vi "LaserCal-Initialize (Dynamic).vi"(0 "Dynamic I-O Params":T1={"Vcommand"="1:0.5:3", "Repeats"=0, "Scramble"=FALSE}, 5 "Taverage (ms)":dbl, 11 "error in (no error)":errorcluster) -> (2 "Stimulus":T4, 4 "Runtime State":T3={"AO Channels"=[], "Fs (Hz)"=100000.0, "Npts"=1}, 8 "SeqVars":dbl[](array[numeric]), 14 "I-O Data":T2, 15 "error out":errorcluster)   [LabVIEW 2015]
uses:
  Typedefs/LaserCal-Stimulus Params.ctl
  Typedefs/LaserCal-Meter Runtime State.ctl
  Typedefs/LaserCal-Data (Dynamic).ctl
  Typedefs/LaserCal-Dynamic I-O Params.ctl
  <vilib>/Analysis/1siggen.llb/Riffle Array (DBL).vi
  <vilib>/Analysis/NI_AALBase.lvlib
panel:
  in  "Fs (Hz)":dbl=100000.0
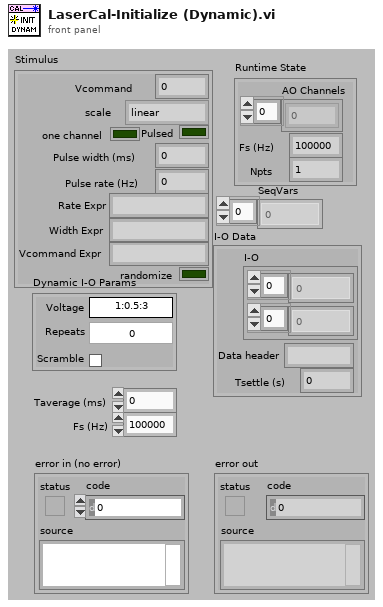
[diagram p1: front panel]
types:
  T1 = typedef "LaserCal-Dynamic I-O Params.ctl" = cluster{"Vcommand":string, "Repeats":i32, "Scramble":bool}
  T2 = typedef "LaserCal-Data (Dynamic).ctl" = cluster{"I-O":cluster{dbl[], dbl[]}, "Data header":string, "Tsettle (s)":dbl}
  T3 = typedef "LaserCal-Meter Runtime State.ctl" = cluster{"AO Channels":i32[], "Fs (Hz)":dbl, "Npts":i32}
  T4 = typedef "LaserCal-Stimulus Params.ctl" = cluster{"Vcommand":dbl, "scale":enum16{"linear", "dB"}, "Pulsed":bool, "Pulse width (ms)":dbl, "Pulse rate (Hz)":dbl, "Vcommand Expr":string, "Width Expr":string, "one channel":bool, "Rate Expr":string, "randomize":bool}
  T5 = cluster{cluster{"Riffled {X}":dbl[], dbl[]}, "Header out":string, "Taverage (ms)":dbl}
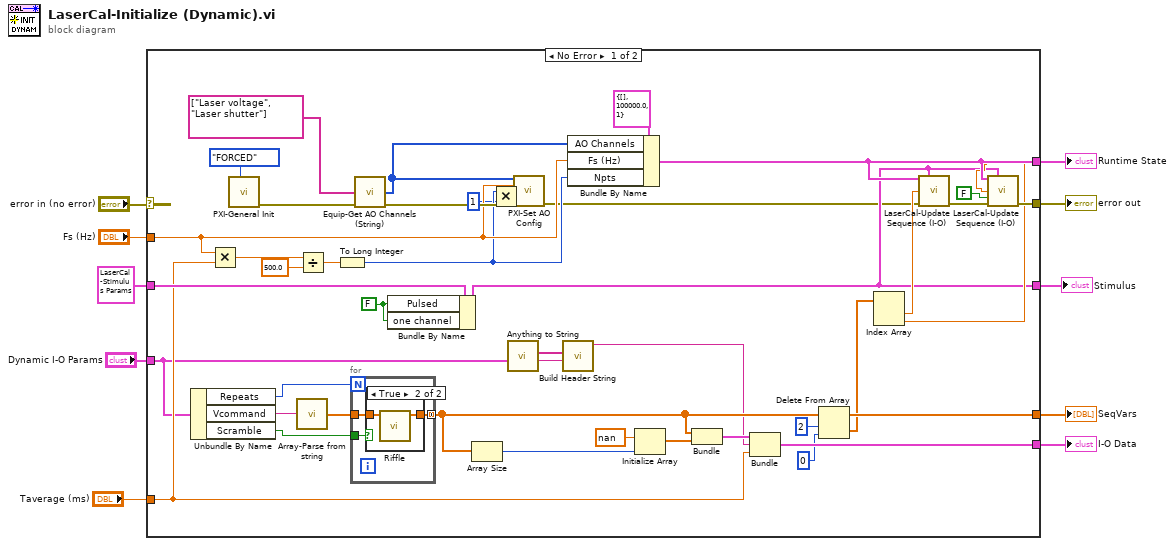
[diagram p0: block diagram]
diagram:
  n1 = case shown="No Error" "error in (no error)" {
    selector: "error in (no error)" -> [_ w59]
    tunnel: [w24 w59] -> w9
    tunnel: "Fs (Hz)" -> [w45 _]
    tunnel: T4 {"Vcommand"=0.0, "scale"=enum."linear", "Pulsed"=FALSE, "Pulse width (ms)"=0.0, "Pulse rate (Hz)"=0.0, "Vcommand Expr"="", "Width Expr"="", "one channel"=FALSE, "Rate Expr"="", "randomize"=FALSE} ("Stimulus") -> [w37 _]
    tunnel: [w23 _] -> w7
    tunnel: [w29 _] -> w6
    tunnel: "Taverage (ms)" -> [w35 _]
    tunnel: [w38 _] -> w4
    tunnel: "Dynamic I-O Params" -> [w13 _]
    tunnel: [w19 _] -> w2
    frame No Error {
      w11 = FALSE ("Pulsed")
      n2 = Unbundle By Name(w13) -> ("Repeats"=w17:i32, "Vcommand"=w43:string, "Scramble"=w18:bool)
      n3 = Multiply(x=w45, y=w35) -> (x*y=w48:dbl)
      n4 = call "PXI-General Init.vi"("Double Buffer Mode"=enum32{"OFF", "ENABLED", "FORCED"}."FORCED") -> ("error out"=w51:errorcluster)  [unwired: 10 in]
      n5 = call "Array-Parse from string.vi"("String"=w43) -> ("Array"=w36:dbl[])  [unwired: 13 in, 1 out]
      n6 = Divide(x=w48, y=500.0) -> (x/y=w34:dbl)
      n7 = To Long Integer(number=w34) -> (32bit integer=w44:i32)
      n8 = for {
        N: w17 -> [_]
        tunnel: w36 -> [w55]
        tunnel: [w54] -> w32 mode=concatenating
        tunnel: w18 -> [w53]
        n9 = case shown="True" w53 {
          tunnel: w55 -> [w56 w58]
          tunnel: [w56 w57] -> w54
          frame False {
          }
          frame True {
            n10 = call-poly <vilib>:"Riffle.vi"("X"=w58) -> ("Riffled {X}"=w57:dbl[])  [unwired: 8 in, 2 out]
          }
        }
      }
      n11 = call "Equip-Get AO Channels (String).vi"("Channel Names"=string[] ["Laser voltage", "Laser shutter"], "error in (no error)"=w51) -> ("AO Channels"=w46:i32[], "error out"=w50:errorcluster)  [unwired: 12 in]
      n12 = Bundle By Name(cluster=w37, "Pulsed"=w11, "one channel"=w11) -> (w19:T4)
      n13 = Array Size(array=w32) -> (size(s)=w41:i32)
      n14 = Multiply(x=w44, y=1) -> (x*y=w27:i32)
      n15 = call "Anything to String.vi"("Anything"=w13) -> ("Section"=w14:string, "Strings[]"=w15:string[])  [unwired: 8 in, 1 out]
      n16 = call "PXI-Set AO Config.vi"("AO Channels"=w46, "Sampling Rate (Hz)"=w45, "Buffer Size"=w27, "error in (no error)"=w50) -> ("error out"=w16:errorcluster)  [unwired: 11 in]
      n17 = call "Build Header String.vi"("Section"=w14, "Strings[]"=w15) -> ("Header out"=w12:string)  [unwired: 9 in]
      n18 = Bundle By Name(cluster=T3 {"AO Channels"=[], "Fs (Hz)"=100000.0, "Npts"=1} ("Runtime State"), "AO Channels"=w46, "Fs (Hz)"=w45, "Npts"=w44) -> (w23:T3)
      n19 = Initialize Array(nan ("element"), w41) -> (w40:dbl[])
      n20 = Bundle("Riffled {X}"=w32, w40) -> (w39:cluster{"Riffled {X}":dbl[], dbl[]})  [unwired: 1 in]
      n21 = Bundle(w39, "Header out"=w12, "Taverage (ms)"=w35) -> (w38:T5)  [unwired: 1 in]
      n22 = Delete From Array(array=w32, length=2, index=0) -> (deleted portion=w28:dbl[], array with subset deleted=w29:dbl[])
      n23 = Index Array(array=w28) -> (element #1=w30:dbl, element #2=w22:dbl)  [unwired: 2 in]
      n24 = call "LaserCal-Update Sequence (I-O).vi"("Runtime State"=w23, "Stimulus (I-O)"=w19, "SeqVal"=w30, "error in (no error)"=w16) -> ("error out"=w25:errorcluster)  [unwired: 11 in]
      n25 = call "LaserCal-Update Sequence (I-O).vi"("Runtime State"=w23, "Stimulus (I-O)"=w19, "SeqVal"=w22, "Start?"=FALSE, "error in (no error)"=w25) -> ("error out"=w24:errorcluster)  [unwired: 10 in]
    }
    frame Error {
    }
  }
  "error out" <- w9
  "Stimulus" <- w2
  "Runtime State" <- w7
  "SeqVars" <- w6
  "I-O Data" <- w4
